vi "G#Object_RegisterClassAttributes.vi"(0 "reference in":refnum<class "G#Object.lvclass">, 1 "static attribute ref":u32, 5 "error in (no error)":errorcluster) -> (14 "reference out":refnum<class "G#Object.lvclass">, 19 "error out":errorcluster)   [LabVIEW 2017, in "G#Object.lvclass"]
doc: "Registers the object to the G# all objects lists. It also sends an event to the debugger and the desktop trace."
uses:
  <vilib>/addons/_AddQ/G#Object/G#Object.lvclass
  <vilib>/addons/_AddQ/G#Object/utils/G#Object_ObjectInfoType.ctl
  <vilib>/addons/_AddQ/G#Object/utils/G#Object_CreateMethod.ctl
  <vilib>/addons/_AddQ/G#Object/utils/G#Object_EventType.ctl
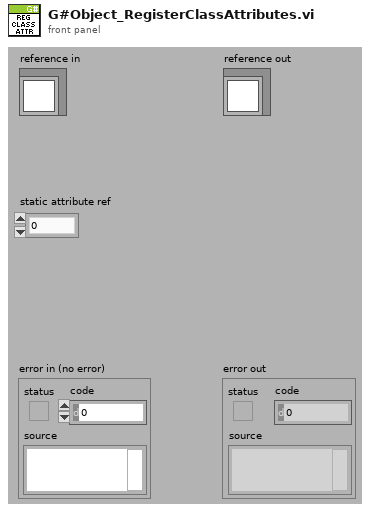
[diagram p1: front panel]
types:
  T1 = typedef "G#Object.lvclass/G#Object_EventType.ctl" = enum16{"Created new", "Looked up existing", "Deleted", "Forced delete", "Not deleted", "Garbage collected", "Cleared", "User", "Error", "External create object", "External create class attributes", "Created class attributes", "Run constructor", "Run constructor done", "Run open method", "Run open method done"}
  T2 = typedef "G#Object.lvclass/G#Object_ObjectInfoType.ctl" = cluster{"ObjectName":string, "ObjectID":u32, "Users":i32, "Counter":bool, "AttributeRefs":u32[], "FullClassName":string, "ClassName":string, "CreateMethod":T3, "GenericDestructorExists":bool, "Owner":string}
  T3 = typedef "G#Object.lvclass/G#Object_CreateMethod.ctl" = enum16{"Create", "Create or look up existing", "Look up existing"}
  T4 = cluster{"full class name":string, "reference in":refnum<class "G#Object.lvclass">}
  T5 = cluster{"full class name":string, "reference in":refnum<class "G#Object.lvclass">}[]
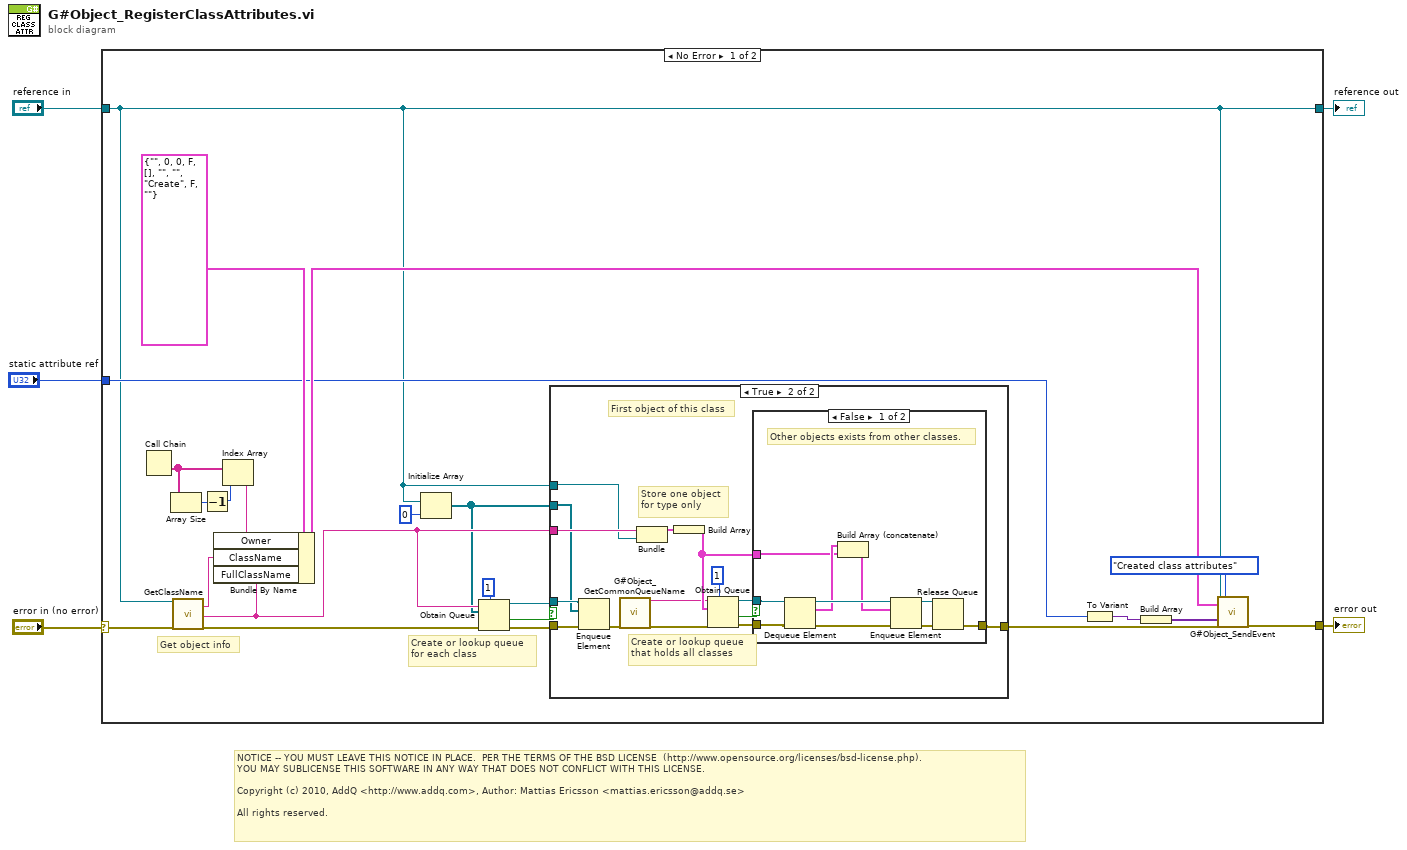
[diagram p0: block diagram]
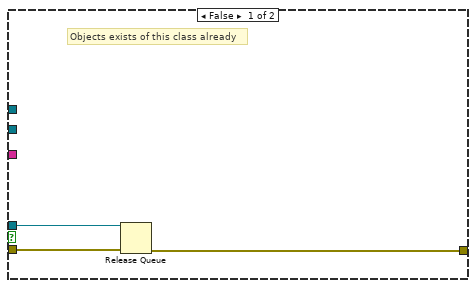
[diagram p2: hidden frame]
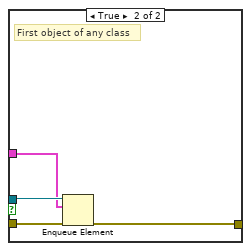
[diagram p3: hidden frame]
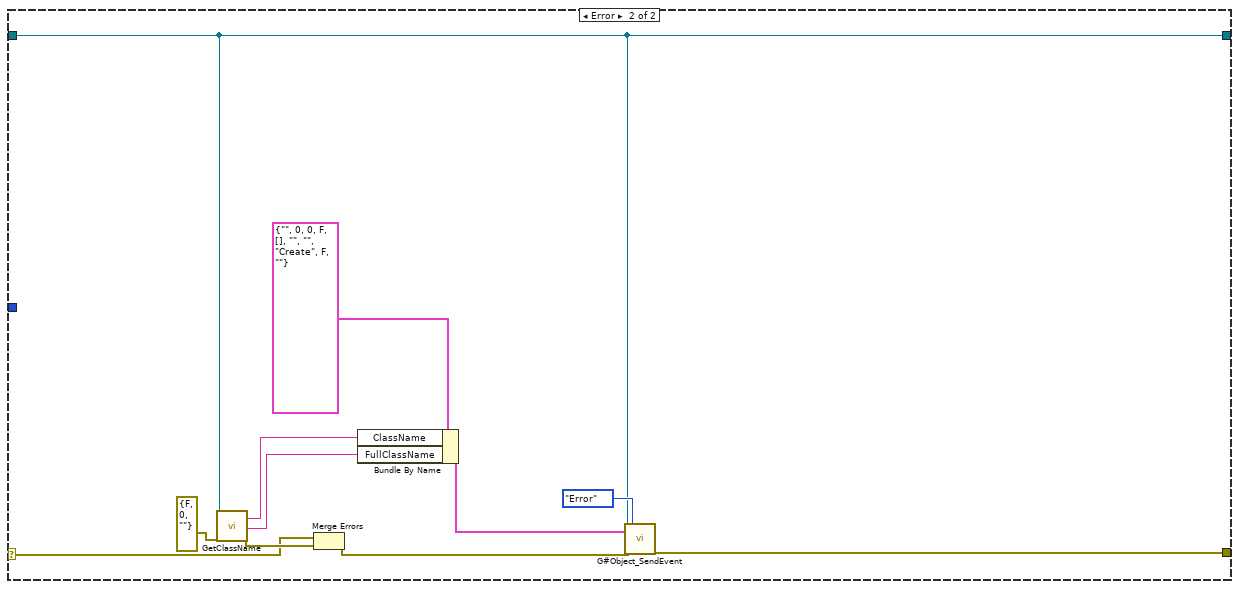
[diagram p4: hidden frame]
diagram:
  # "NOTICE -- YOU MUST LEAVE THIS NOTICE IN PLACE.  PER THE TERMS OF THE BSD LICENSE  (http://www.opensource.org/licenses/bsd-license.php).\nYOU MAY SUBLICENSE THIS SOFTWARE IN ANY WAY THAT DOES NOT CONFLICT WITH THIS LICENSE.\n\nCopyright (c) 2010, AddQ <http://www.addq.com>, Author: Mattias Ericsson <mattias.ericsson@addq.se>\n\nAll rights reserved."
  n1 = case shown="No Error" "error in (no error)" {
    selector: "error in (no error)" -> [w22 w63]
    tunnel: [w23 w71] -> w4
    tunnel: [w12 w61] -> w2
    tunnel: "reference in" -> [w12 w61]
    tunnel: "static attribute ref" -> [w16 _]
    frame No Error {
      # "Get object info"
      # "Create or lookup queue\nfor each class"
      n2 = Call Chain() -> (call chain=w10:string[])
      n3 = Array Size(array=w10) -> (size(s)=w8:i32)
      n4 = call-dynamic "GetClassName.vi"("reference in"=w12, "error in (no error)"=w22) -> ("class name"=w19:string, "full class name"=w18:string, "error out"=w6:errorcluster)  [unwired: 13 in, 2 out]
      n5 = Decrement(x=w8) -> (x-1=w9:i32)
      n6 = Index Array(array=w10, index=w9) -> (element=w7:string)
      n7 = Bundle By Name(cluster=T2 {"ObjectName"="", "ObjectID"=0, "Users"=0, "Counter"=FALSE, "AttributeRefs"=[], "FullClassName"="", "ClassName"="", "CreateMethod"=enum."Create", "GenericDestructorExists"=FALSE, "Owner"=""} ("element"), "Owner"=w7, "ClassName"=w19, "FullClassName"=w18) -> (w20:T2)
      n8 = Initialize Array(w12, 0 ("dimension size")) -> (w13:refnum<class "G#Object.lvclass">[])
      n9 = Obtain Queue(max queue size (-1, unlimited)=1, name (unnamed)=w18, element data type=w13, error in (no error)=w6) -> (queue out=w25:refnum<queue>, created new?=w26:bool, error out=w27:errorcluster)  [unwired: 1 in]
      n10 = case shown="True" w26 {
        tunnel: w27 -> [w31 w37]
        tunnel: w25 -> [w30 w36]
        tunnel: w13 -> [_ w35]
        tunnel: [w29 w46] -> w24
        tunnel: w18 -> [_ w40]
        tunnel: w12 -> [_ w38]
        frame False {
          # "Objects exists of this class already"
          n11 = Release Queue(queue=w30, error in (no error)=w31) -> (error out=w29:errorcluster)  [unwired: 1 in, 2 out]
        }
        frame True {
          # "Store one object\nfor type only"
          # "Create or lookup queue\nthat holds all classes"
          # "First object of this class"
          n12 = Enqueue Element(queue=w36, element=w35, error in (no error)=w37) -> (error out=w34:errorcluster)  [unwired: 1 in, 2 out]
          n13 = call <vilib>:"G#Object_GetCommonQueueName.vi"("error in (no error)"=w34) -> ("queue name"=w32:string, "error out"=w33:errorcluster)  [unwired: 17 in]
          n14 = Bundle("full class name"=w40, "reference in"=w38) -> (w39:T4)  [unwired: 1 in]
          n15 = Build Array(w39) -> (w42:T5)
          n16 = Obtain Queue(max queue size (-1, unlimited)=1, name (unnamed)=w32, element data type=w42, error in (no error)=w33) -> (queue out=w44:refnum<queue>, created new?=w43:bool, error out=w45:errorcluster)  [unwired: 1 in]
          n17 = case shown="False" w43 {
            tunnel: w45 -> [w51 w60]
            tunnel: [w56 w59] -> w46
            tunnel: w44 -> [w50 w58]
            tunnel: w42 -> [w52 w57]
            frame False {
              # "Other objects exists from other classes."
              n18 = Dequeue Element(queue=w50, error in (no error)=w51) -> (queue out=w55:refnum<queue>, element=w53:T5, error out=w49:errorcluster)  [unwired: 1 in, 1 out]
              n19 = Build Array (concatenate)(w53, w52) -> (w54:T5)
              n20 = Enqueue Element(queue=w55, element=w54, error in (no error)=w49) -> (queue out=w47:refnum<queue>, error out=w48:errorcluster)  [unwired: 1 in, 1 out]
              n21 = Release Queue(queue=w47, error in (no error)=w48) -> (error out=w56:errorcluster)  [unwired: 1 in, 2 out]
            }
            frame True {
              # "First object of any class"
              n22 = Enqueue Element(queue=w58, element=w57, error in (no error)=w60) -> (error out=w59:errorcluster)  [unwired: 1 in, 2 out]
            }
          }
        }
      }
      n23 = To Variant(anything=w16) -> (Variant=w15:variant)
      n24 = Build Array(w15) -> (w14:variant[])
      n25 = call <vilib>:"G#Object_SendEvent.vi"("reference in"=w12, "object info extended"=w20, "parameters"=w14, "error in (no error)"=w24, "G# event type"=G#Object_EventType."Created class attributes" ("G#Event")) -> ("error out"=w23:errorcluster)  [unwired: 14 in]
    }
    frame Error {
      n26 = call-dynamic "GetClassName.vi"("reference in"=w61, "error in (no error)"=errorcluster {"status"=FALSE, "code"=0, "source"=""}) -> ("class name"=w66:string, "full class name"=w65:string, "error out"=w69:errorcluster)  [unwired: 13 in, 2 out]
      n27 = Merge Errors(w63, w69) -> (w62:errorcluster)
      n28 = Bundle By Name(cluster=T2 {"ObjectName"="", "ObjectID"=0, "Users"=0, "Counter"=FALSE, "AttributeRefs"=[], "FullClassName"="", "ClassName"="", "CreateMethod"=enum."Create", "GenericDestructorExists"=FALSE, "Owner"=""}, "ClassName"=w66, "FullClassName"=w65) -> (w64:T2)
      n29 = call <vilib>:"G#Object_SendEvent.vi"("reference in"=w61, "object info extended"=w64, "error in (no error)"=w62, "G# event type"=G#Object_EventType."Error") -> ("error out"=w71:errorcluster)  [unwired: 15 in]
    }
  }
  "error out" <- w4
  "reference out" <- w2
